vi "Export_Clipboard.vi"(5 "Clipboard":refnum<vi>, 7 "Is Copy? (F)":bool, 8 "error in":errorcluster, 11 "Data in":T1={"Class"={"Ants"=refnum, "Layer"=refnum, "Templates"=refnum, "Icon"=refnum, "Glyph"=refnum, "Settings"=refnum, "Tools"=refnum}, "Ref"={"Add Layer"=refnum, "Remove Layer"=refnum, "Line Text"=[], "Body Text Spec"=refnum, "DNL_Font"=refnum, "glyph path str"=refnum, "templates path str"=refnum, "Arrow Up"=refnum, "Arrow Down"=refnum, "IE VI Ref"=refnum, "Glyphs tree"=refnum, "Templates tree"=refnum, "Layer Icon Text"=refnum, "Layer Template"=refnum, "Body Text"=refnum, "Search Templates"=refnum, "TextMarker"=refnum, "Tab Control"=refnum, "Search Glyphs"=refnum, "Line Color"=refnum, "DNL_Glyphs []"=refnum, "Fill Color"=refnum, "Tools"=refnum, "Icon"=refnum, "Preview"=refnum, "Ants"=refnum, "Terminals"=refnum, "menu reference"=refnum, "LayerNames"=[], "GlyphLoadAnimation"=refnum, "TemplateLoadAnimation"=refnum, "refreshGlyphs"=refnum, "refreshTemplates"=refnum}, "Support"={"AntsRect"={"left"=0, "top"=0, "right"=0, "bottom"=0}, "Mouse Move Coords"={"Horizontal"=0, "Vertical"=0}, "Mouse Down Coords"={"Horizontal"=0, "Vertical"=0}, "Temp Coord"={"Horizontal"=0, "Vertical"=0}, "Action"=enum."Default", "Edge Color"=4914962, "Fill Color"=16860, "Mouse Down?"=FALSE, "Draft Mode?"=FALSE, "Temp Icon"=bytes[3102], "CTRL Pressed"=FALSE, "Move Selection?"=FALSE, "AntsRect Orig"={"left"=0, "top"=0, "right"=0, "bottom"=0}, "Text"="", "TM Set?"=FALSE, "Mouse inside icon?"=FALSE, "Tool (old value)"=0, "Pencil Move Color"=0, "Swap Colors?"=FALSE, "Shift pressed?"=FALSE}}) -> (0 "error out":errorcluster)   [LabVIEW 2021]
doc: "Saves selection image to the clipboard."
uses:
  <resource>/plugins/NIIconEditor/Controls/Global Data.ctl
  <resource>/plugins/NIIconEditor/Class/Ants/Ants.lvclass
  <resource>/plugins/NIIconEditor/Class/FakedArray/FakedArray.lvclass
  <vilib>/LabVIEW Icon API/lv_icon/Classes/Icon/Icon.lvclass
  <resource>/plugins/NIIconEditor/Class/Icon Library/Glyph.lvclass
  <resource>/plugins/NIIconEditor/Class/Settings/Settings.lvclass
  <resource>/plugins/NIIconEditor/Class/Tools/Tools Paint.lvclass
  <resource>/plugins/NIIconEditor/Controls/IE Classes.ctl
  <resource>/plugins/NIIconEditor/Controls/References Cluster.ctl
  <resource>/plugins/NIIconEditor/Controls/SupportClass.ctl
  <vilib>/Utility/miscctls.llb/LVPoint32TypeDef.ctl
  <resource>/plugins/NIIconEditor/Controls/SupportClass_Action.ctl
  <vilib>/LabVIEW Icon API/lv_icon/Controls/IEColor.ctl
  <vilib>/Utility/miscctls.llb/LVBoundsTypeDef.ctl
  <vilib>/LabVIEW Icon API/lv_icon/Classes/Icon Framework/Icon Framework.lvclass
  C:/Users/J63553/Projects/_LabVIEW Community/labview-icon-editor/vi.lib/LabVIEW Icon API/lv_icon/Classes/Layer/Layer.lvclass
  <vilib>/LabVIEW Icon API/lv_icon/lv_icon.lvlib
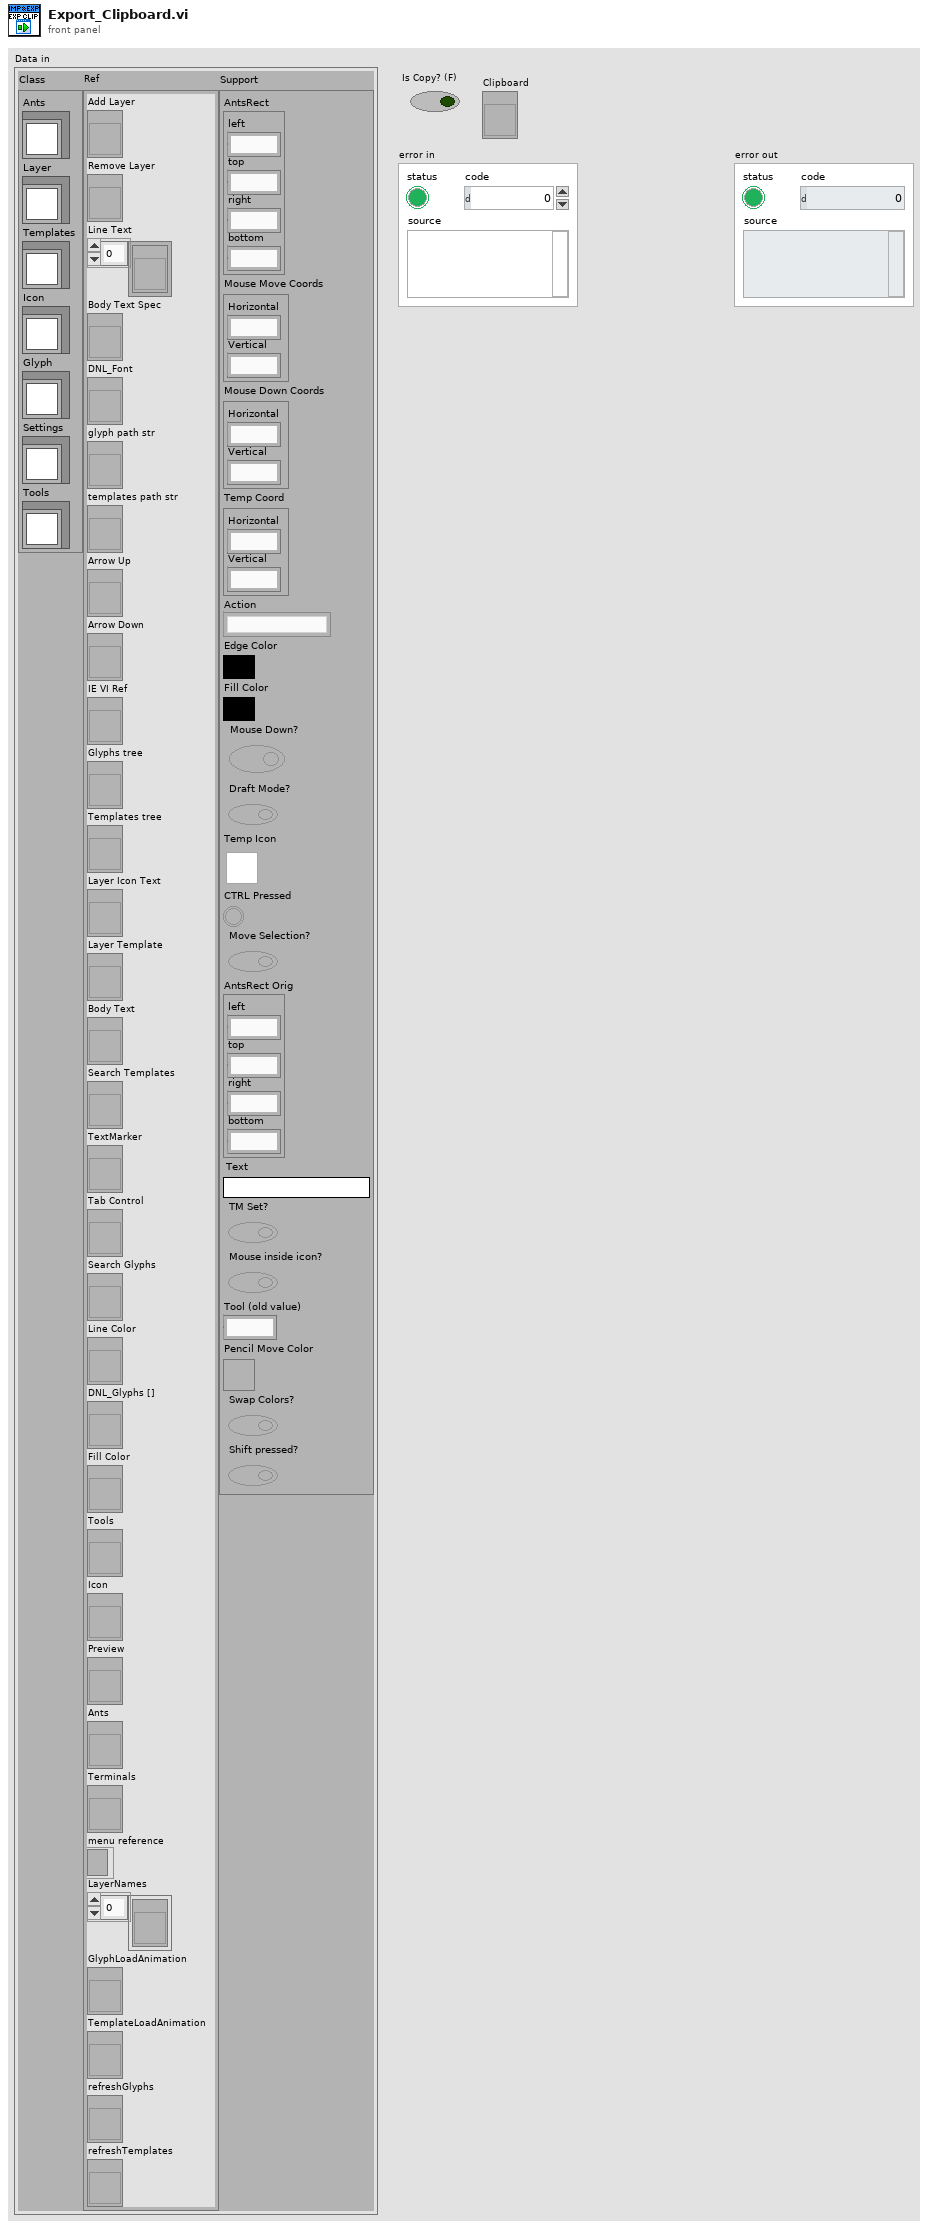
[diagram p1: front panel]
types:
  T1 = typedef "lv_icon.lvlib/Global Data.ctl" = cluster{"Class":T2, "Ref":T3, "Support":T4}
  T2 = typedef "IE Classes.ctl" = cluster{"Ants":refnum<class "Ants.lvclass">, "Layer":refnum<class "FakedArray.lvclass">, "Templates":refnum<class "FakedArray.lvclass">, "Icon":refnum<class "Icon.lvclass">, "Glyph":refnum<class "Glyph.lvclass">, "Settings":refnum<class "Settings.lvclass">, "Tools":refnum<class "Tools Paint.lvclass">}
  T3 = typedef "lv_icon.lvlib/References Cluster.ctl" = cluster{"Add Layer":refnum<vi>, "Remove Layer":refnum<vi>, "Line Text":refnum<vi>[], "Body Text Spec":refnum<vi>, "DNL_Font":refnum<vi>, "glyph path str":refnum<vi>, "templates path str":refnum<vi>, "Arrow Up":refnum<vi>, "Arrow Down":refnum<vi>, "IE VI Ref":refnum<vi>, "Glyphs tree":refnum<vi>, "Templates tree":refnum<vi>, "Layer Icon Text":refnum<vi>, "Layer Template":refnum<vi>, "Body Text":refnum<vi>, "Search Templates":refnum<vi>, "TextMarker":refnum<vi>, "Tab Control":refnum<vi>, "Search Glyphs":refnum<vi>, "Line Color":refnum<vi>, "DNL_Glyphs []":refnum<vi>, "Fill Color":refnum<vi>, "Tools":refnum<vi>, "Icon":refnum<vi>, "Preview":refnum<vi>, "Ants":refnum<vi>, "Terminals":refnum<vi>, "menu reference":refnum<k9>, "LayerNames":refnum<vi>[], "GlyphLoadAnimation":refnum<vi>, "TemplateLoadAnimation":refnum<vi>, "refreshGlyphs":refnum<vi>, "refreshTemplates":refnum<vi>}
  T4 = typedef "SupportClass.ctl" = cluster{"AntsRect":cluster{"left":i16, "top":i16, "right":i16, "bottom":i16}, "Mouse Move Coords":T5, "Mouse Down Coords":T5, "Temp Coord":T5, "Action":T6, "Edge Color":T7, "Fill Color":T7, "Mouse Down?":bool, "Draft Mode?":bool, "Temp Icon":picture, "CTRL Pressed":bool, "Move Selection?":bool, "AntsRect Orig":cluster{"left":i16, "top":i16, "right":i16, "bottom":i16}, "Text":string, "TM Set?":bool, "Mouse inside icon?":bool, "Tool (old value)":u32, "Pencil Move Color":u32, "Swap Colors?":bool, "Shift pressed?":bool}
  T5 = typedef "LVPoint32TypeDef.ctl" = cluster{"Horizontal":i32, "Vertical":i32}
  T6 = typedef "SupportClass_Action.ctl" = enum16{"Default", "Move Selection", "Glyph Library", "Tool"}
  T7 = typedef "IEColor.ctl" = u32
  T8 = typedef "LVBoundsTypeDef.ctl" = cluster{"Width":u32, "Height":u32}
  T9 = cluster{"left":i16, "top":i16, "right":i16, "bottom":i16}
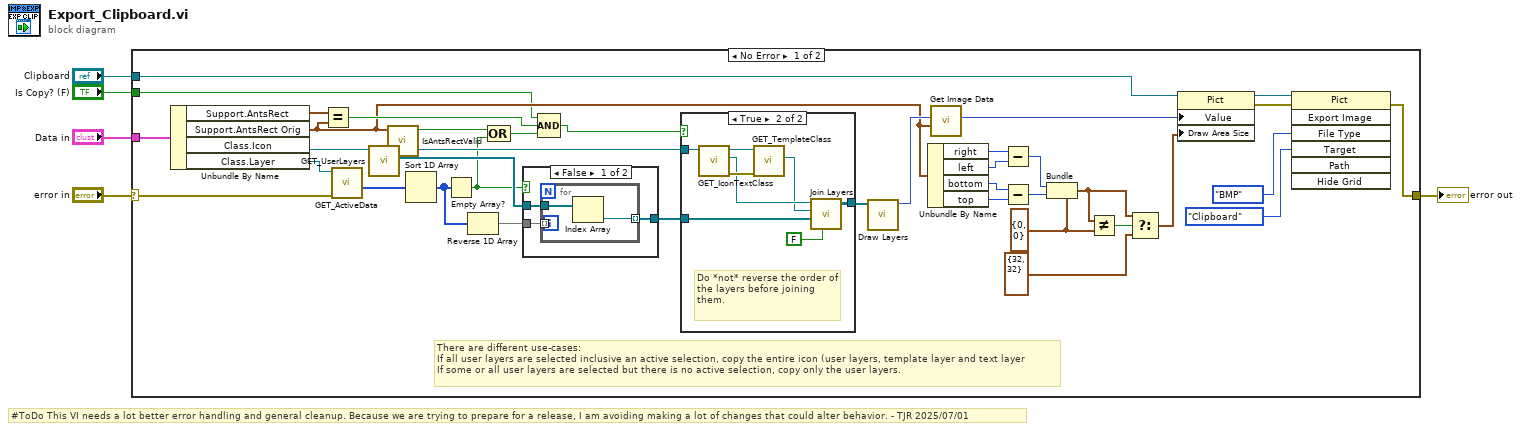
[diagram p0: block diagram]
diagram:
  # "#ToDo This VI needs a lot better error handling and general cleanup. Because we are trying to prepare for a release, I am avoiding making a lot of changes that could alter behavior. - TJR 2025/07/01"
  n1 = case shown="No Error" "error in" {
    selector: "error in" -> [w41 w59]
    tunnel: [w42 w59] -> w4
    tunnel: "Data in" -> [w20 _]
    tunnel: "Is Copy? (F)" -> [w10 _]
    tunnel: "Clipboard" -> [w9 _]
    frame No Error {
      w8 = T8 {"Width"=0, "Height"=0} ("Draw Area Size")
      # "There are different use-cases:\nIf all user layers are selected inclusive an active selection, copy the entire icon (user layers, template layer and text layer\nIf some or all user layers are selected but there is no active selection, copy only the user layers."
      n2 = Unbundle By Name(w20) -> ("Support.AntsRect"=w13:T9, "Support.AntsRect Orig"=w12:T9, "Class.Icon"=w18:refnum<class "Icon.lvclass">, "Class.Layer"=w19:refnum<class "FakedArray.lvclass">)
      n3 = Equal?(x=w13, y=w12) -> (x = y?=w15:bool)
      n4 = call-dynamic "GET_ActiveData.vi"("error in (no error)"=w41, "FakedArray in"=w19) -> ("Active Data []"=w28:i32[])  [unwired: 9 out]
      n5 = call-dynamic "GET_UserLayers.vi"("Icon.lvclass in"=w18) -> ("All Layers"=w29:refnum<class "Layer.lvclass">[], "Icon.lvclass out"=w23:refnum<class "Icon.lvclass">)  [unwired: 1 in, 8 out]
      n6 = call <resource>:"IsAntsRectValid.vi"("AntsRect"=w12) -> ("Valid?"=w21:bool)  [unwired: 10 out]
      n7 = Sort 1D Array(array=w28) -> (sorted array=w27:i32[])
      n8 = Empty Array?(array=w27) -> (empty?=w11:bool)
      n9 = Reverse 1D Array(array=w27) -> (reversed array=w26:i32[])
      n10 = Compound Arithmetic op=OR(w21, w11) -> (w16:bool)
      n11 = case shown="False" w11 {
        tunnel: w29 -> [w55 w58]
        tunnel: [w54 w58] -> w22
        tunnel: w26 -> [w53 _]
        frame False {
          n12 = for {
            tunnel: w55 -> [w57]
            tunnel: w53 -> [_] mode=indexing
            tunnel: [w56] -> w54 mode=indexing
            n13 = Index Array(array=w57) -> (element=w56:refnum<class "Layer.lvclass">)  [unwired: 1 in]
          }
        }
        frame True {
        }
      }
      n14 = Compound Arithmetic op=AND(w10, w15, w16) -> (w14:bool)
      n15 = case shown="True" w14 {
        tunnel: w23 -> [_ w50]
        tunnel: [w44 w49] -> w17
        tunnel: w22 -> [w44 w46]
        frame False {
        }
        frame True {
          # "Do *not* reverse the order of the layers before joining them."
          n16 = call-dynamic "GET_IconTextClass.vi"("Icon.lvclass in"=w50) -> ("error out"=w52:errorcluster, "Icon Framework.lvclass"=w48:refnum<class "Icon Framework.lvclass">, "Icon.lvclass out"=w51:refnum<class "Icon.lvclass">)  [unwired: 1 in, 7 out]
          n17 = call-dynamic "GET_TemplateClass.vi"("error in (no error)"=w52, "Icon.lvclass in"=w51) -> ("Icon Framework.lvclass"=w47:refnum<class "Icon Framework.lvclass">)  [unwired: 9 out]
          n18 = call <vilib>:"Join Layers.vi"("Rotate? (T)"=FALSE, "User Layers"=w46, "Template"=w47, "Icon Text"=w48) -> ("Layer out"=w49:refnum<class "Layer.lvclass">[])  [unwired: 2 in, 5 out]
        }
      }
      n19 = call <vilib>:"Draw Layers.vi"("Layers"=w17) -> ("Picture"=w30:picture)  [unwired: 4 in, 6 out]
      n20 = Unbundle By Name(w12) -> ("right"=w40:i16, "left"=w39:i16, "bottom"=w38:i16, "top"=w37:i16)
      n21 = call <vilib>:"Get Image Data.vi"("subset rect"=w12, "Pic In"=w30) -> ("Pic Out"=w31:picture)  [unwired: 1 in, 8 out]
      n22 = Subtract(x=w40, y=w39) -> (x-y=w35:i16)
      n23 = Subtract(x=w38, y=w37) -> (x-y=w36:i16)
      n24 = Bundle(cluster=w8, "Width"=w35, "Height"=w36) -> (w24:T8)
      n25 = Not Equal?(x=w24, y=w8) -> (x != y?=w25:bool)
      n26 = Select(t=w24, s=w25, f=T8 {"Width"=32, "Height"=32} ("Draw Area Size")) -> (s? t:f=w6:T8)
      n27 = property on="Property Node" class="Pict"(reference=w9, "Value"=w31, "Draw Area Size"=w6) -> (reference out=w32:refnum<vi>, error out=w43:errorcluster)  [unwired: 1 in]
      n28 = invoke on="Invoke Node" class="Pict" method="Export Image"(reference=w32, error in=w43, "File Type"=enum32{"BMP", "EPS", "EMF", "PICT"}."BMP", "Target"=enum32{"File", "Clipboard"}."Clipboard") -> (error out=w42:errorcluster)  [unwired: 3 in, 6 out]
    }
    frame Error {
    }
  }
  "error out" <- w4
